vi "DIO 입출력.vi"() -> ()   [LabVIEW 2019]
uses:
  <vilib>/Utility/error.llb/DialogType.ctl
  <vilib>/DAQmx/write.llb/DAQmx Write (Digital 1D Bool 1Chan 1Samp).vi
  <vilib>/DAQmx/read.llb/DAQmx Read (Digital 1D Bool 1Chan 1Samp).vi
  <vilib>/DAQmx/create/channels.llb/DAQmx Create Channel (DI-Digital Input).vi
  <vilib>/DAQmx/miscellaneous.llb/DAQmx Fill In Error Info.vi
  <vilib>/DAQmx/create/channels.llb/DAQmx Create Channel (DO-Digital Output).vi
panel:
  in  "data 2":bool[](array[boolean]) caption="데이터"
  out "data":bool[](array[boolean]) caption="데이터"
  in  "라인 3":tag="Dev1/port0/line0:1"
  in  "정지 2":bool
  in  "루프 시간 (ms) 2":u32=100
  in  "라인":tag="Dev1/port0/line0:1"
  in  "정지":bool
  in  "루프 시간 (ms)":u32=100
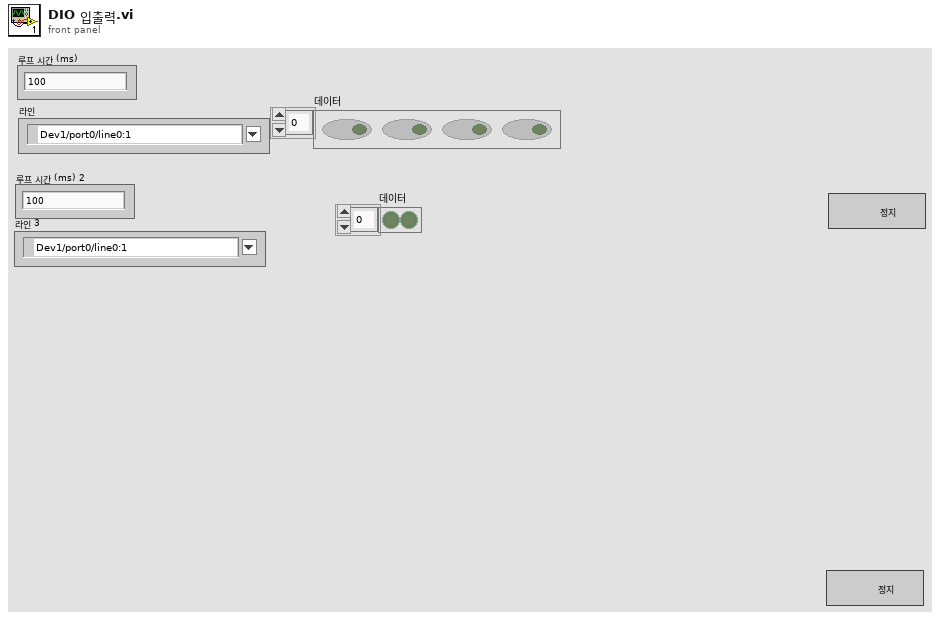
[diagram p1: front panel]
types:
  T1 = typedef "DialogType.ctl" = u16
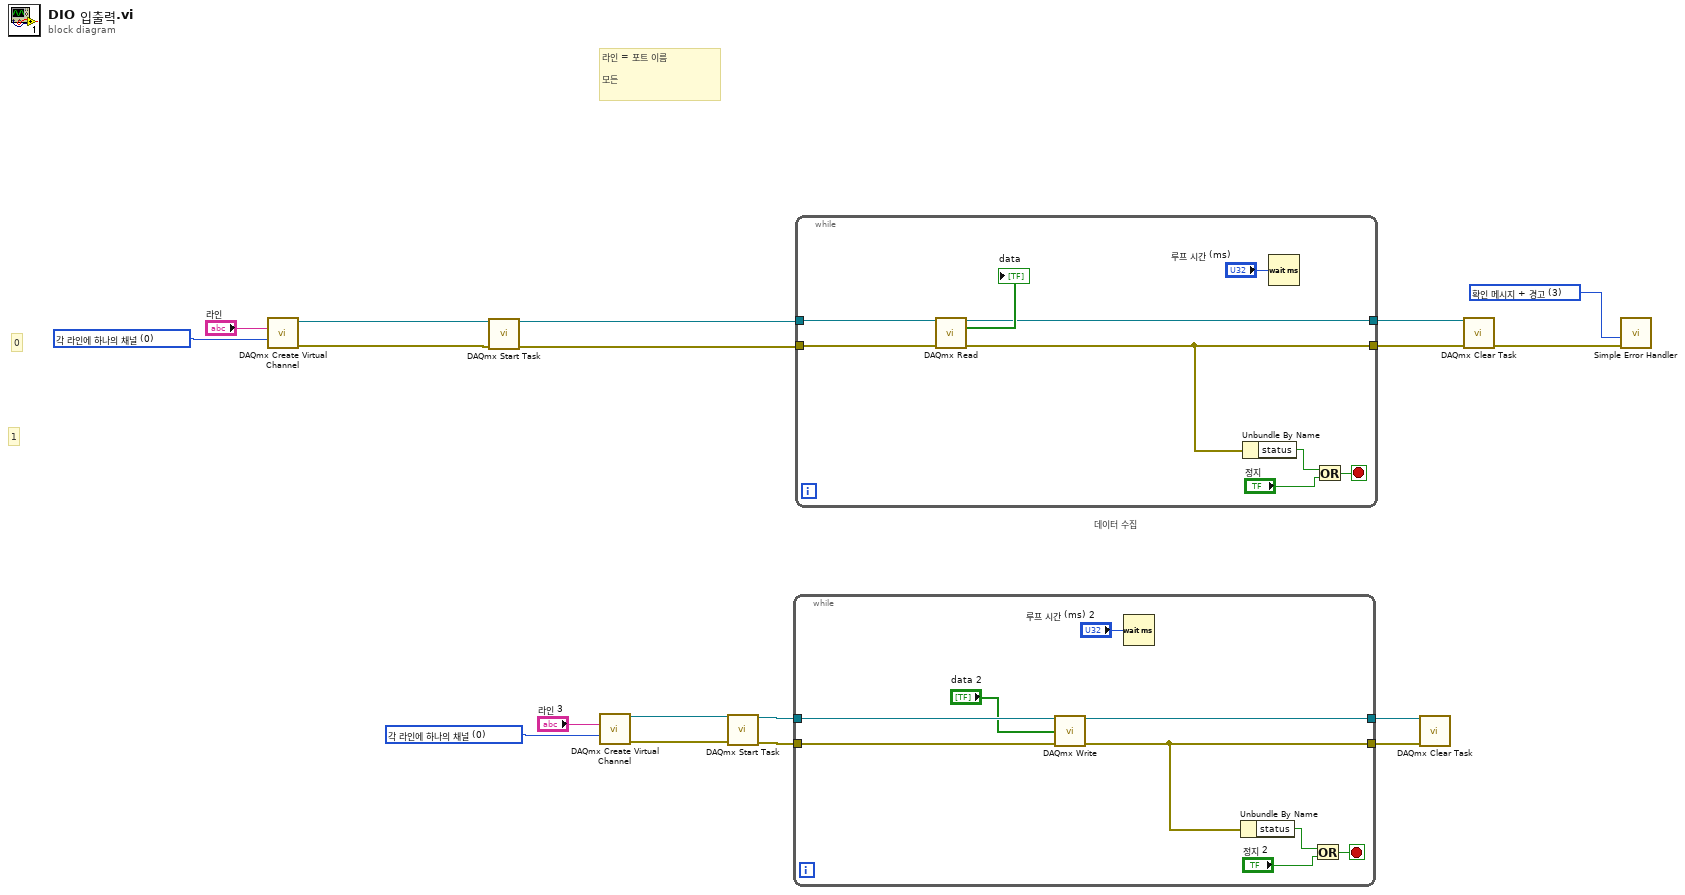
[diagram p0: block diagram]
diagram:
  w14 = 0 items=["각 라인에 하나의 채널", "모든 라인에 하나의 채널"] ("line grouping")
  w15 = 0 items=["각 라인에 하나의 채널", "모든 라인에 하나의 채널"] ("line grouping")
  w16 = T1 3 items=["대화 상자 없음", "확인 메시지", "메시지 지속 또는 정지", "확인 메시지 + 경고", "지속/정지 + 경고"] ("대화 상자 타입 (확인 메시지:1)")
  # "1"
  # "0"
  # "라인 = 포트 이름   \n\n모든"
  # "데이터 수집"
  n1 = call-poly <vilib>:"DAQmx Create Virtual Channel.vi"("lines"="라인", "line grouping"=w15) -> ("task out"=w8:refnum<k21>, "error out"=w7:errorcluster)  [unwired: 12 in]
  n2 = call <vilib>:"DAQmx Start Task.vi"("task/channels in"=w8, "error in"=w7) -> ("task out"=w6:refnum<k21>, "error out"=w5:errorcluster)  [unwired: 12 in]
  n3 = call-poly <vilib>:"DAQmx Create Virtual Channel.vi"("lines"="라인 3", "line grouping"=w14) -> ("task out"=w12:refnum<k21>, "error out"=w11:errorcluster)  [unwired: 12 in]
  n4 = call <vilib>:"DAQmx Start Task.vi"("task/channels in"=w12, "error in"=w11) -> ("task out"=w10:refnum<k21>, "error out"=w9:errorcluster)  [unwired: 12 in]
  n5 = while {
    tunnel: w10 -> [w24]
    tunnel: w9 -> [w23]
    tunnel: [w22] -> w2
    tunnel: [w21] -> w1
    stop <- w27 stop-if-true
    n6 = call-poly <vilib>:"DAQmx Write.vi"("task/channels in"=w24, "data"="data 2", "error in"=w23) -> ("task out"=w22:refnum<k21>, "error out"=w21:errorcluster)  [unwired: 10 in, 1 out]
    n7 = Wait (ms)(milliseconds to wait="루프 시간 (ms) 2") -> ()  [unwired: 1 out]
    n8 = Unbundle By Name(w21) -> ("status"=w20:bool)
    n9 = Or(x=w20, y="정지 2") -> (x .or. y?=w27:bool)
  }
  n10 = while {
    tunnel: w6 -> [w33]
    tunnel: w5 -> [w32]
    tunnel: [w30] -> w4
    tunnel: [w29] -> w3
    stop <- w36 stop-if-true
    n11 = call-poly <vilib>:"DAQmx Read.vi"("task/channels in"=w33, "error in"=w32) -> ("task out"=w30:refnum<k21>, "data"=→"data":bool[], "error out"=w29:errorcluster)  [unwired: 11 in]
    n12 = Unbundle By Name(w29) -> ("status"=w28:bool)
    n13 = Wait (ms)(milliseconds to wait="루프 시간 (ms)") -> ()  [unwired: 1 out]
    n14 = Or(x=w28, y="정지") -> (x .or. y?=w36:bool)
  }
  n15 = call <vilib>:"DAQmx Clear Task.vi"("task in"=w2, "error in"=w1) -> ()  [unwired: 13 in, 1 out]
  n16 = call <vilib>:"DAQmx Clear Task.vi"("task in"=w4, "error in"=w3) -> ("error out"=w18:errorcluster)  [unwired: 13 in]
  n17 = call <vilib>:"Simple Error Handler.vi"("type of dialog (OK msg:1)"=w16, "error in (no error)"=w18) -> ()  [unwired: 3 in, 5 out]
